vi "HA3_yufan_dong.vi"() -> ()   [LabVIEW 2021]
uses:
  Controls/digital_number_display_yufan_dong.ctl
  <vilib>/DAQmx/read.llb/DAQmx Read (Analog 1D Wfm NChan NSamp).vi
  <vilib>/DAQmx/write.llb/DAQmx Write (Digital 1D Bool 1Chan 1Samp).vi
  <vilib>/DAQmx/create/channels.llb/DAQmx Create Channel (AI-Voltage-Basic).vi
  <vilib>/DAQmx/configure/timing.llb/DAQmx Timing (Sample Clock).vi
  <vilib>/DAQmx/create/channels.llb/DAQmx Create Channel (DO-Digital Output).vi
  <vilib>/DAQmx/miscellaneous.llb/DAQmx Fill In Error Info.vi
  <resource>/objmgr/daqmx.rc
panel:
  out "Meaure Rest":i32 caption="in Queue"
  out "Measring":i32=1 caption="in Progress"
  out "Measure Done":i32 caption="Finished"
  out "Measure Total":i32 caption="Total"
  in  "Wait":bool
  in  "MeasureGoOn":bool
  in  "CountDown":bool
  out "error out":errorcluster
  in  "Output Channel (LEDs)":tag="Dev1/port0/line0:1"
  out "Waveform Graph":waveform(dbl)[](graph)
  in  "Input Channel (AI)":tag="Dev1/ai0"
  out "Current State":string
  out "?":T1
  out "Consumer Delay (ms)":u32
  in  "Stop":bool
  in  "Measure":bool
  # "Note & Guide\n\n<<<<<< Channels >>>>>\nInput Channel\n<device>/ai0:1\neg. myDAQ1/ai0:1\n\nOutput Channel\n<device>/<port>/line0:7\neg. myDAQ1/port0/line0:7\n\n\n<<<<<< Controls >>>>>\nMeasure\nadd a count down phase and a measure phase into the qeueu\n\nStop\nstop in 100ms\n\n\n<<<<<<< Others >>>>>>\nAuthor\nYufan Dong - 14.Oct.2021"
  # "Measuring System with Count Down"
  # "System Information"
  # "Measurement Count"
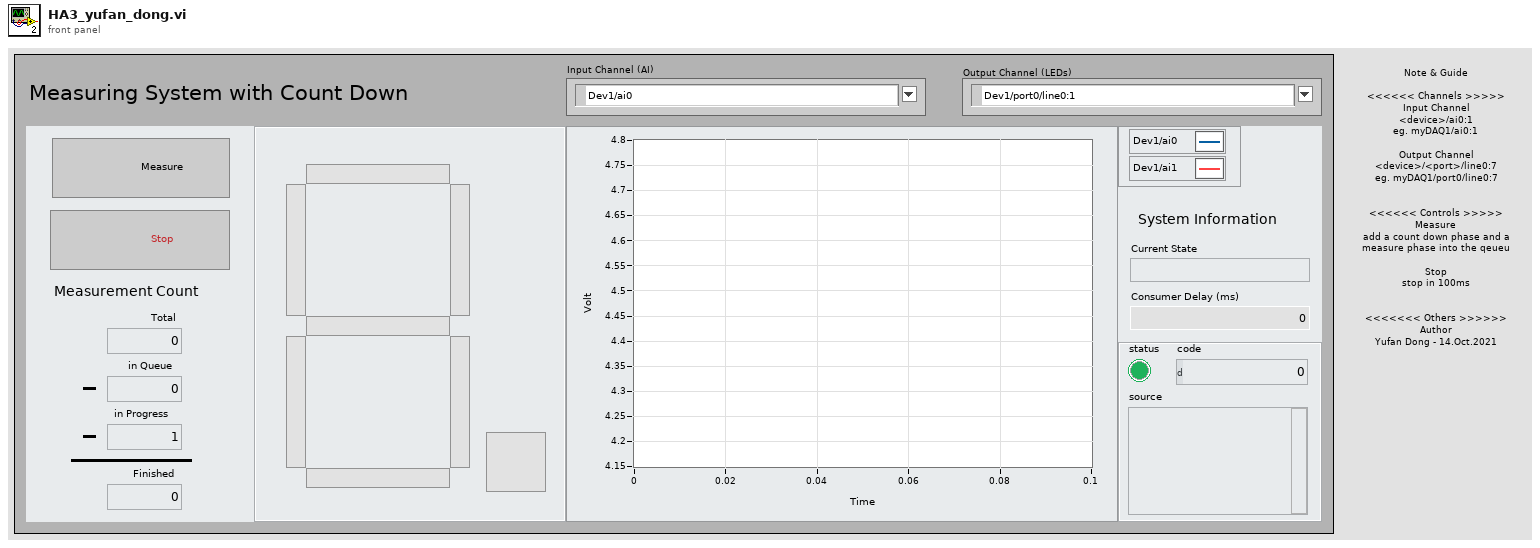
[diagram p1: front panel]
types:
  T1 = typedef "digital_number_display_yufan_dong.ctl" = cluster{"A":bool, "B":bool, "C":bool, "D":bool, "E":bool, "F":bool, "G":bool, "DP":bool}
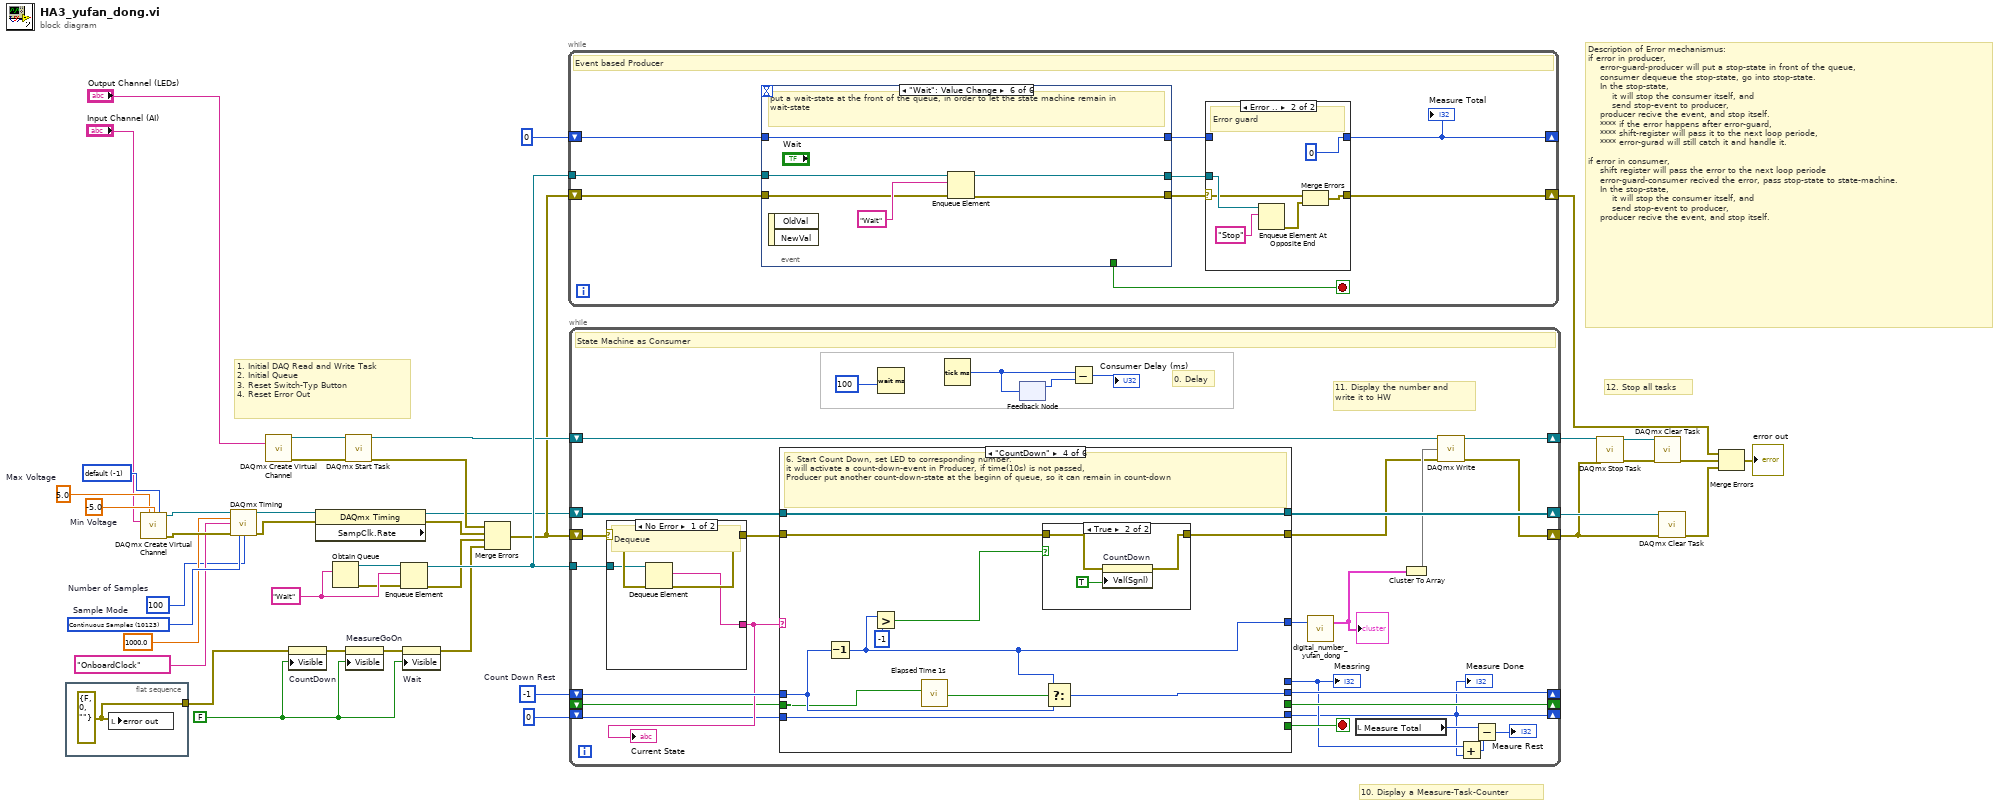
[diagram p0: block diagram]
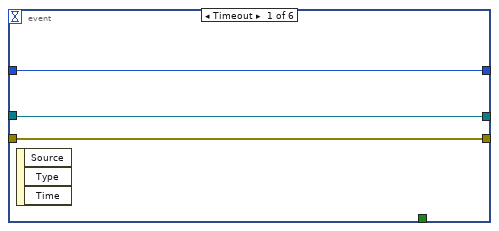
[diagram p3: hidden frame]
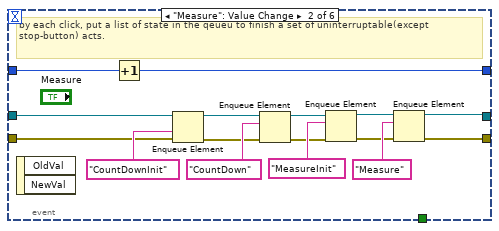
[diagram p4: hidden frame]
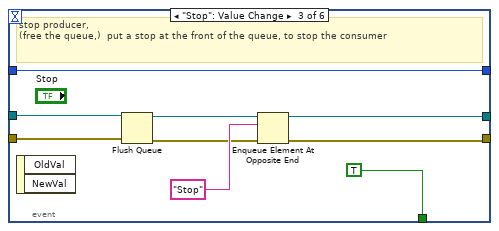
[diagram p5: hidden frame]
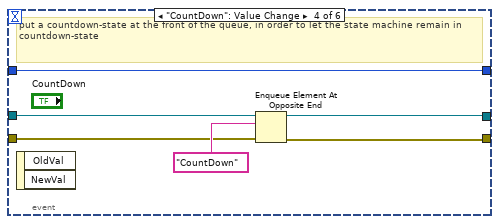
[diagram p6: hidden frame]
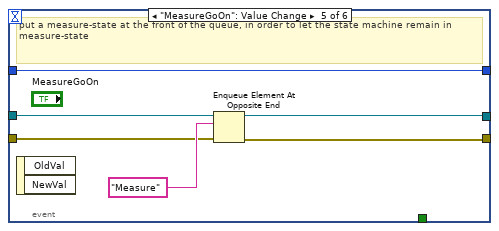
[diagram p7: hidden frame]
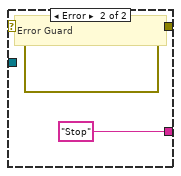
[diagram p8: hidden frame]
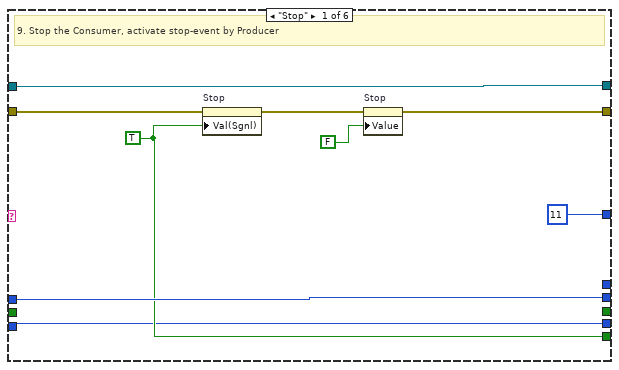
[diagram p9: hidden frame]
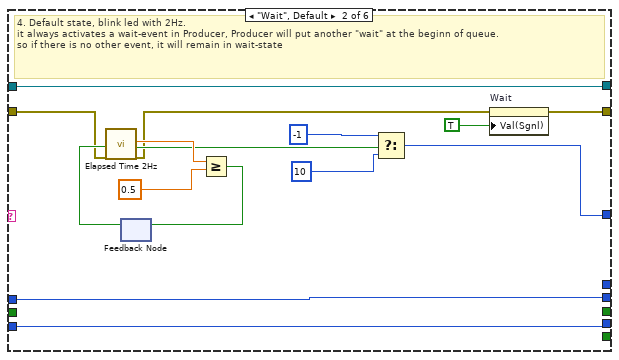
[diagram p10: hidden frame]
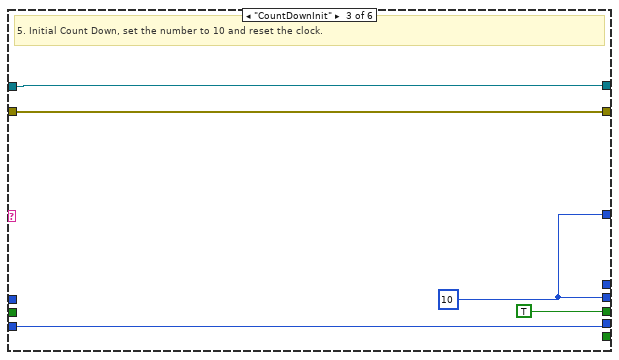
[diagram p11: hidden frame]
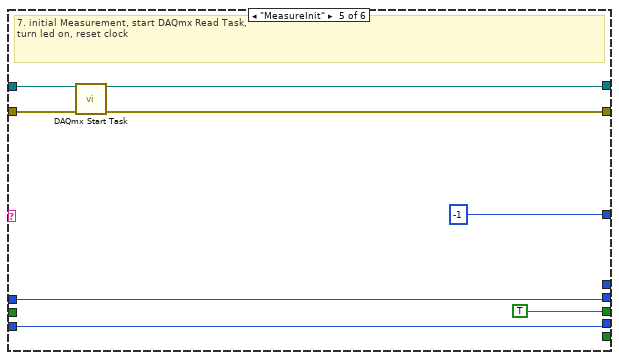
[diagram p13: hidden frame]
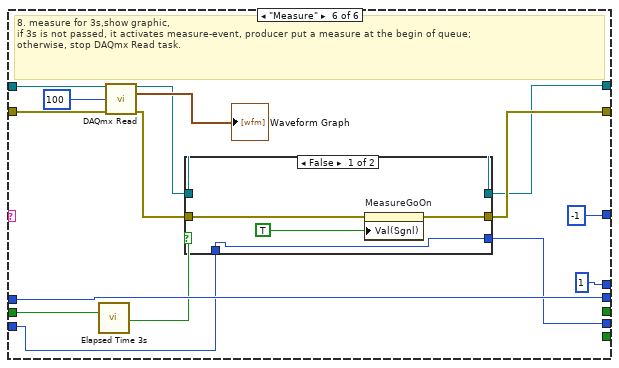
[diagram p14: hidden frame]
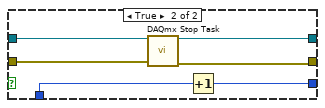
[diagram p15: hidden frame]
diagram:
  w18 = -1  # Count Down Rest
  w31 = -1 items=["default"=-1, "RSE"=10083, "NRSE"=10078, "Differential"=10106, "Pseudodifferential"=12529] ("Terminal Configuration")
  w27 = 100  # Number of Samples
  w32 = 5.0  # Max Voltage
  w33 = -5.0  # Min Voltage
  w37 = 10123 items=["Finite Samples"=10178, "Continuous Samples"=10123, "Hardware Timed Single Point"=12522]  # Sample Mode
  w12 = FALSE
  w41 = "Wait"
  # "Description of Error mechanismus: \nif error in producer, \n    error-guard-producer will put a stop-state in front of the queue, \n    consumer dequeue the stop-state, go into stop-state. \n    In the stop-state, \n        it will stop the consumer itself, and \n        send stop-event to producer, \n    producer recive the event, and stop itself.\n    **** if the error happens after error-guard, \n    **** shift-register will pass it to the next loop periode, \n    **** error-gurad will still catch it and handle it.\n\nif error in consumer,\n    shift register will pass the error to the next loop periode\n    error-guard-consumer recived the error, pass stop-state to state-machine.\n    In the stop-state, \n        it will stop the consumer itself, and \n        send stop-event to producer, \n    producer recive the event, and stop itself."
  # "10. Display a Measure-Task-Counter"
  # "1. Initial DAQ Read and Write Task\n2. Initial Queue\n3. Reset Switch-Typ Button\n4. Reset Error Out"
  # "12. Stop all tasks"
  n1 = flat-sequence {
    tunnel: [w43] -> w1
    frame #0 {
      w43 = errorcluster {"status"=FALSE, "code"=0, "source"=""} ("error out")
      n2 = local write "error out"(w43) -> ()
    }
  }
  n3 = call-poly <vilib>:"DAQmx Create Virtual Channel.vi"("maximum value"=w32, "minimum value"=w33, "input terminal configuration"=w31, "physical channels"="Input Channel (AI)") -> ("task out"=w35:refnum<k21>, "error out"=w36:errorcluster)  [unwired: 10 in]
  n4 = call-poly <vilib>:"DAQmx Timing.vi"("task/channels in"=w35, "sample mode"=w37, "samples per channel"=w27, "rate"=1000.0 ("Sample Rate"), "source"=tag "OnboardClock" ("Sample Clock Source"), "error in"=w36) -> ("task out"=w38:refnum<k21>, "error out"=w28:errorcluster)  [unwired: 8 in]
  n5 = call-poly <vilib>:"DAQmx Create Virtual Channel.vi"("lines"="Output Channel (LEDs)") -> ("task out"=w25:refnum<k21>, "error out"=w26:errorcluster)  [unwired: 13 in]
  n6 = property on="CountDown" class="Bool (strict)"(error in=w1, "Visible"=w12) -> (error out=w6:errorcluster)  [unwired: 1 in, 1 out]
  n7 = property class="DAQmx Timing" props=["SampClk.Rate"](reference=w38, error in=w28) -> (reference out=w11:refnum<k21>, error out=w8:errorcluster)  [unwired: 1 out]
  n8 = Obtain Queue(element data type=w41) -> (queue out=w42:refnum<queue>, error out=w40:errorcluster)  [unwired: 4 in, 1 out]
  n9 = call <vilib>:"DAQmx Start Task.vi"("task/channels in"=w25, "error in"=w26) -> ("task out"=w23:refnum<k21>, "error out"=w19:errorcluster)  [unwired: 12 in]
  n10 = property on="MeasureGoOn" class="Bool (strict)"(error in=w6, "Visible"=w12) -> (error out=w5:errorcluster)  [unwired: 1 in, 1 out]
  n11 = Enqueue Element(queue=w42, element=w41, error in (no error)=w40) -> (queue out=w39:refnum<queue>, error out=w7:errorcluster)  [unwired: 1 in, 1 out]
  n12 = property on="Wait" class="Bool (strict)"(error in=w5, "Visible"=w12) -> (error out=w4:errorcluster)  [unwired: 1 in, 1 out]
  n13 = Merge Errors(w19, w8, w7, w4) -> (w17:errorcluster)
  n14 = while {
    tunnel: w39 -> [w52]
    shift-right: [w48] -> w16
    shift-left: w17 -> [w50]
    shift-right: [w44] -> _
    shift-left: 0 -> [w46]
    stop <- w51 stop-if-true
    # "Event based Producer"
    n15 = event shown="[5] \"Wait\": Value Change" {
      selector: _ -> [_ _ _ _ _ _]
      dyn-events: _ -> [_ _ _ _ _ _]
      timeout: _ -> [_ _ _ _ _ _]
      tunnel: w52 -> [w62 w79 w87 w93 w99 w105]
      tunnel: [_ _ TRUE _ _ _] -> w51
      tunnel: w50 -> [w63 w71 w85 w92 w98 w104]
      tunnel: [w63 w67 w83 w90 w97 w103] -> w49
      tunnel: [w62 w66 w82 w91 w96 w102] -> w47
      tunnel: w46 -> [w61 w65 w80 w89 w95 w101]
      tunnel: [w61 w64 w80 w89 w95 w101] -> w45
      event Timeout {
        n16 = event-data() -> ()  [unwired: 1 in, 3 out]
      }
      event "Measure": Value Change {
        # "by each click, put a list of state in the qeueu to finish a set of uninterruptable(except stop-button) acts."
        n17 = event-data() -> ()  [unwired: 1 in, 2 out]
        n18 = Increment(x=w65) -> (x+1=w64:i32)
        n19 = Enqueue Element(queue=w79, element="CountDownInit", error in (no error)=w71) -> (queue out=w76:refnum<queue>, error out=w70:errorcluster)  [unwired: 1 in, 1 out]
        n20 = Enqueue Element(queue=w76, element="CountDown", error in (no error)=w70) -> (queue out=w75:refnum<queue>, error out=w69:errorcluster)  [unwired: 1 in, 1 out]
        n21 = Enqueue Element(queue=w75, element="MeasureInit", error in (no error)=w69) -> (queue out=w72:refnum<queue>, error out=w68:errorcluster)  [unwired: 1 in, 1 out]
        n22 = Enqueue Element(queue=w72, element="Measure", error in (no error)=w68) -> (queue out=w66:refnum<queue>, error out=w67:errorcluster)  [unwired: 1 in, 1 out]
      }
      event "Stop": Value Change {
        # "stop producer, \n(free the queue,)  put a stop at the front of the queue, to stop the consumer"
        n23 = event-data() -> ()  [unwired: 1 in, 2 out]
        n24 = Flush Queue(queue=w87, error in (no error)=w85) -> (queue out=w86:refnum<queue>, error out=w84:errorcluster)  [unwired: 1 out]
        n25 = Enqueue Element At Opposite End(queue=w86, element="Stop", error in (no error)=w84) -> (queue out=w82:refnum<queue>, error out=w83:errorcluster)  [unwired: 1 in, 1 out]
      }
      event "CountDown": Value Change {
        # "put a countdown-state at the front of the queue, in order to let the state machine remain in countdown-state"
        n26 = event-data() -> ()  [unwired: 1 in, 2 out]
        n27 = Enqueue Element At Opposite End(queue=w93, element="CountDown", error in (no error)=w92) -> (queue out=w91:refnum<queue>, error out=w90:errorcluster)  [unwired: 1 in, 1 out]
      }
      event "MeasureGoOn": Value Change {
        # "put a measure-state at the front of the queue, in order to let the state machine remain in measure-state"
        n28 = event-data() -> ()  [unwired: 1 in, 2 out]
        n29 = Enqueue Element At Opposite End(queue=w99, element="Measure", error in (no error)=w98) -> (queue out=w96:refnum<queue>, error out=w97:errorcluster)  [unwired: 1 in, 1 out]
      }
      event "Wait": Value Change {
        # "put a wait-state at the front of the queue, in order to let the state machine remain in wait-state"
        n30 = event-data() -> ()  [unwired: 1 in, 2 out]
        n31 = Enqueue Element(queue=w105, element="Wait", error in (no error)=w104) -> (queue out=w102:refnum<queue>, error out=w103:errorcluster)  [unwired: 1 in, 1 out]
      }
    }
    n32 = case shown="Error .." w49 {
      selector: w49 -> [w54 w58]
      tunnel: [w54 w57] -> w48
      tunnel: w47 -> [_ w59]
      tunnel: w45 -> [w53 _]
      tunnel: [w53 0] -> w44
      frame No Error {
      }
      frame Error {
        # "Error guard"
        n33 = Enqueue Element At Opposite End(queue=w59, element="Stop") -> (error out=w56:errorcluster)  [unwired: 2 in, 2 out]
        n34 = Merge Errors(w58, w56) -> (w57:errorcluster)
      }
    }
    "Measure Total" <- w44
  }
  n35 = while {
    tunnel: w39 -> [w116]
    shift-right: [w130] -> _
    shift-left: w18 -> [w131]
    shift-right: [w113] -> w9
    shift-left: w17 -> [w115]
    shift-right: [w120] -> _
    shift-left: _ -> [w119]
    shift-right: [w117] -> w10
    shift-left: w11 -> [w118]
    shift-right: [w124] -> w20
    shift-left: w23 -> [w126]
    shift-right: [w107] -> _
    shift-left: 0 -> [w112]
    stop <- w122 stop-if-true
    # "11. Display the number and \nwrite it to HW"
    # "0. Delay"
    # "State Machine as Consumer"
    n36 = case shown="No Error" w115 {
      selector: w115 -> [w137 w139]
      tunnel: [w135 "Stop"] -> w121
      tunnel: w116 -> [w136 _]
      tunnel: [w138 w139] -> w114
      frame No Error {
        # "Dequeue"
        n37 = Dequeue Element(queue=w136, error in (no error)=w137) -> (element=w135:string, error out=w138:errorcluster)  [unwired: 1 in, 2 out]
      }
      frame Error {
        # "Error Guard"
      }
    }
    "Current State" <- w121
    n38 = case shown="\"CountDown\"" w121 {
      tunnel: [w147 _ _ _ _ _] -> w122
      tunnel: w131 -> [w149 w164 _ w176 w192 w207]
      tunnel: [w149 w164 w167 w179 w192 w207] -> w130
      tunnel: [11 w159 w167 w175 -1 -1] -> w129
      tunnel: [_ _ TRUE _ TRUE _] -> w120
      tunnel: w114 -> [w143 w155 w169 w174 w187 w198]
      tunnel: [w142 w152 w169 w173 w186 w205] -> w123
      tunnel: w119 -> [_ _ _ w172 _ w204]
      tunnel: w118 -> [w144 w151 w166 w171 w189 w201]
      tunnel: [w144 w151 w166 w171 w188 w199] -> w117
      tunnel: w112 -> [w141 w150 w165 w170 w185 w195]
      tunnel: [w141 w150 w165 w170 w185 w194] -> w107
      tunnel: [_ _ _ _ _ 1] -> w108
      frame "Stop" {
        w147 = TRUE
        # "9. Stop the Consumer, activate stop-event by Producer"
        n39 = property on="Stop" class="Bool (strict)"(error in=w143, "Val(Sgnl)"=w147) -> (error out=w145:errorcluster)  [unwired: 1 in, 1 out]
        n40 = property on="Stop" class="Bool (strict)"(error in=w145, "Value"=FALSE) -> (error out=w142:errorcluster)  [unwired: 1 in, 1 out]
      }
      frame "Wait", Default {
        # "4. Default state, blink led with 2Hz. \nit always activates a wait-event in Producer, Producer will put another \"wait\" at the beginn of queue. \nso if there is no other event, it will remain in wait-state"
        n41 = feedback #1() -> (w160:bool)  [unwired: 1 in]
        n42 = call "Elapsed Time 2Hz"("Auto Reset"=w160, "error in (no error)"=w155) -> ("Elapsed Time (s)"=w163:dbl, "Time has Elapsed"=w158:bool, "error out"=w153:errorcluster)  [unwired: 10 in, 5 out]
        n43 = Greater Or Equal?(x=w163, y=0.5) -> (x >= y?=w161:bool)
        n44 = feedback-in #1(w161) -> ()
        n45 = Select(t=-1, s=w158, f=10) -> (s? t:f=w159:i32)
        n46 = property on="Wait" class="Bool (strict)"(error in=w153, "Val(Sgnl)"=TRUE) -> (error out=w152:errorcluster)  [unwired: 1 in, 1 out]
      }
      frame "CountDownInit" {
        w167 = 10
        # "5. Initial Count Down, set the number to 10 and reset the clock."
      }
      frame "CountDown" {
        # "6. Start Count Down, set LED to corresponding number.\nit will activate a count-down-event in Producer, if time(10s) is not passed, \nProducer put another count-down-state at the beginn of queue, so it can remain in count-down"
        n47 = Decrement(x=w176) -> (x-1=w175:i32)
        n48 = Greater?(x=w175, y=-1) -> (0:w177:bool)
        n49 = call "Elapsed Time 1s"("Reset"=w172) -> ("Time has Elapsed"=w180:bool)  [unwired: 11 in, 7 out]
        n50 = case shown="True" w177 {
          tunnel: w174 -> [w181 w183]
          tunnel: [w181 w182] -> w173
          frame False {
          }
          frame True {
            n51 = property on="CountDown" class="Bool (strict)"(error in=w183, "Val(Sgnl)"=TRUE) -> (error out=w182:errorcluster)  [unwired: 1 in, 1 out]
          }
        }
        n52 = Select(t=w175, s=w180, f=w176) -> (s? t:f=w179:i32)
      }
      frame "MeasureInit" {
        # "7. initial Measurement, start DAQmx Read Task, \nturn led on, reset clock"
        n53 = call <vilib>:"DAQmx Start Task.vi"("task/channels in"=w189, "error in"=w187) -> ("task out"=w188:refnum<k21>, "error out"=w186:errorcluster)  [unwired: 12 in]
      }
      frame "Measure" {
        # "8. measure for 3s,show graphic,\nif 3s is not passed, it activates measure-event, producer put a measure at the begin of queue;\notherwise, stop DAQmx Read task."
        n54 = call "Elapsed Time 3s"("Reset"=w204) -> ("Time has Elapsed"=w203:bool)  [unwired: 11 in, 7 out]
        n55 = call-poly <vilib>:"DAQmx Read.vi"("task/channels in"=w201, "number of samples per channel"=100, "error in"=w198) -> ("task out"=w200:refnum<k21>, "data"=→"Waveform Graph":waveform(dbl)[], "error out"=w196:errorcluster)  [unwired: 10 in]
        n56 = case shown="False" w203 {
          tunnel: w196 -> [w211 w216]
          tunnel: [w210 w215] -> w205
          tunnel: w200 -> [w209 w218]
          tunnel: [w209 w217] -> w199
          tunnel: w195 -> [w208 w214]
          tunnel: [w208 w213] -> w194
          frame False {
            n57 = property on="MeasureGoOn" class="Bool (strict)"(error in=w211, "Val(Sgnl)"=TRUE) -> (error out=w210:errorcluster)  [unwired: 1 in, 1 out]
          }
          frame True {
            n58 = call <vilib>:"DAQmx Stop Task.vi"("task/channels in"=w218, "error in"=w216) -> ("task out"=w217:refnum<k21>, "error out"=w215:errorcluster)  [unwired: 12 in]
            n59 = Increment(x=w214) -> (x+1=w213:i32)
          }
        }
      }
    }
    "Measure Done" <- w107
    "Measring" <- w108
    n60 = Wait (ms)(milliseconds to wait=u32 100) -> ()  [unwired: 1 out]
    n61 = Tick Count (ms)() -> (millisecond timer value=w133:u32)
    n62 = feedback #2() -> (w134:u32)  [unwired: 1 in]
    n63 = feedback-in #2(w133) -> ()
    n64 = Subtract(x=w133, y=w134) -> (x-y=→"Consumer Delay (ms)":u32)
    n65 = call "digital_number_yufan_dong.vi"("Numeric Control"=w129) -> ("Digital"=w127:T1)  [unwired: 2 in]
    "?" <- w127
    n66 = local read "Measure Total"() -> (w110:i32)
    n67 = Cluster To Array(cluster=w127) -> (array=w125:bool[])
    n68 = call-poly <vilib>:"DAQmx Write.vi"("task/channels in"=w126, "data"=w125, "error in"=w123) -> ("task out"=w124:refnum<k21>, "error out"=w113:errorcluster)  [unwired: 10 in, 1 out]
    n69 = Add(x=w108, y=w107) -> (x+y=w111:i32)
    n70 = Subtract(x=w110, y=w111) -> (x-y=→"Meaure Rest":i32)
  }
  n71 = call <vilib>:"DAQmx Stop Task.vi"("task/channels in"=w20, "error in"=w9) -> ("task out"=w22:refnum<k21>, "error out"=w21:errorcluster)  [unwired: 12 in]
  n72 = call <vilib>:"DAQmx Clear Task.vi"("task in"=w22, "error in"=w21) -> ("error out"=w15:errorcluster)  [unwired: 13 in]
  n73 = call <vilib>:"DAQmx Clear Task.vi"("task in"=w10, "error in"=w9) -> ("error out"=w14:errorcluster)  [unwired: 13 in]
  n74 = Merge Errors(w16, w15, w14) -> (→"error out":errorcluster)
